vi "Get Boolean.vi"(8 "error in (no error)":errorcluster, 11 "BooleanMessage in":refnum<class "BooleanMessage.lvclass">) -> (0 "error out":errorcluster, 2 "Message Data":bool, 3 "BooleanMessage out":refnum<class "BooleanMessage.lvclass">)   [LabVIEW 2009, in "LapDog.Messaging.v2.NativeTypes.lvlib" / "BooleanMessage.lvclass"]
doc: "Returns the data contained in the message.\n\nThis method executes regardless of the error in state."
uses:
  BooleanMessage.lvclass
  BooleanMessage.lvclass/BooleanMessage.ctl
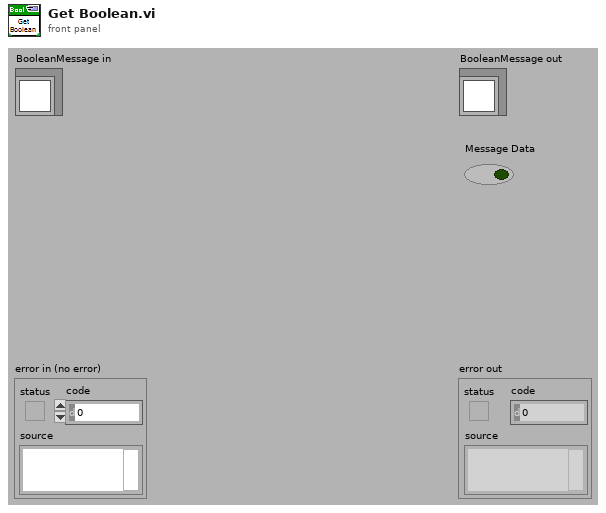
[diagram p1: front panel]
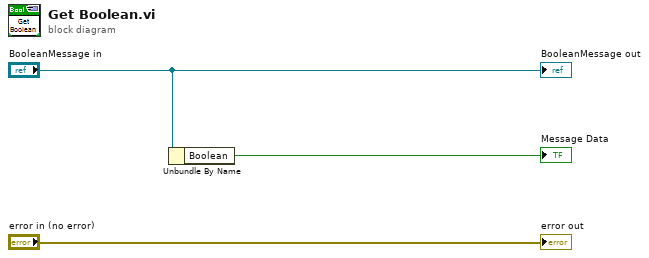
[diagram p0: block diagram]
diagram:
  n1 = Unbundle By Name("BooleanMessage in") -> ("Boolean"=→"Message Data":bool)
  "error out" <- "error in (no error)"
  "BooleanMessage out" <- "BooleanMessage in"
